vi "ManualAutoScan.vi"(8 "Button-OK":bool, 10 "menu reference":refnum<k9>, 11 "SN Length":string) -> (1 "MainProcess":T1, 3 "Barcode out:":string)   [LabVIEW 2013]
uses:
  Control/SystemProcess.ctl
  Control/Buffer.vi
panel:
  in  "menu reference 2":refnum<k9>
  in  "Button-Cancel":bool
  in  "Barcode(S/N):":string
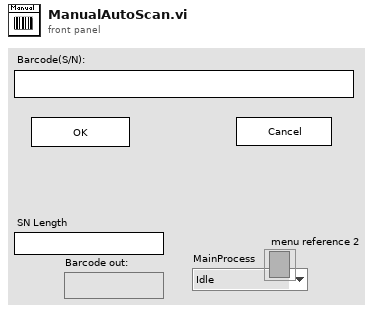
[diagram p1: front panel]
types:
  T1 = typedef "SystemProcess.ctl" = enum16{"Idle", "SystemInit", "SpecialEvent", "Barcode(SN)", "TestInitialize", "Test", "Stop", "SaveTestData", "Exit"}
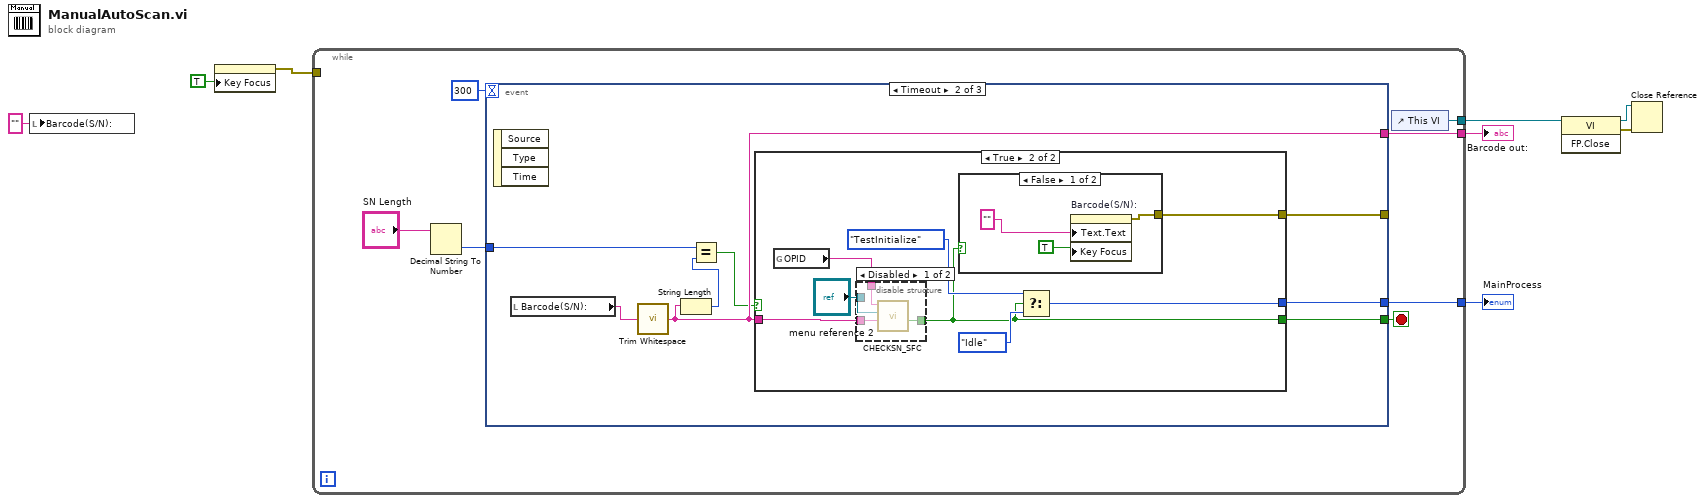
[diagram p0: block diagram]
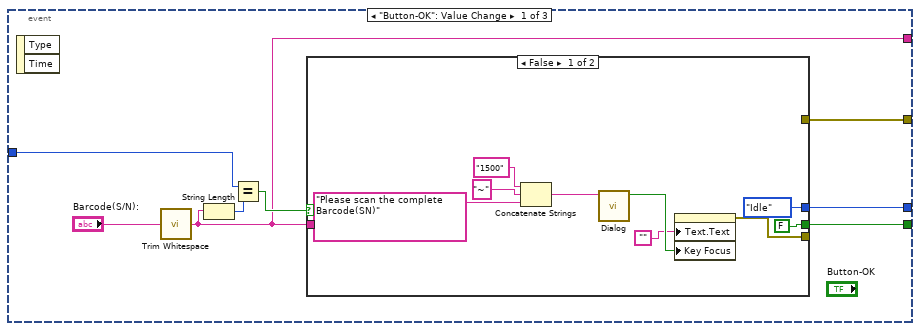
[diagram p2: hidden frame]
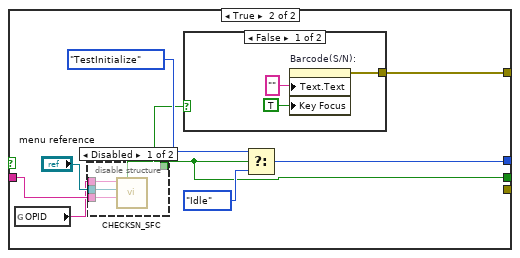
[diagram p3: hidden frame]
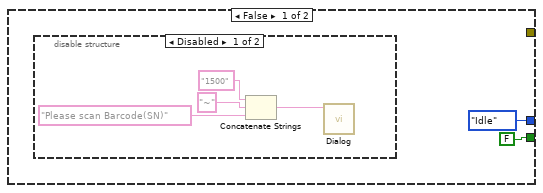
[diagram p6: hidden frame]
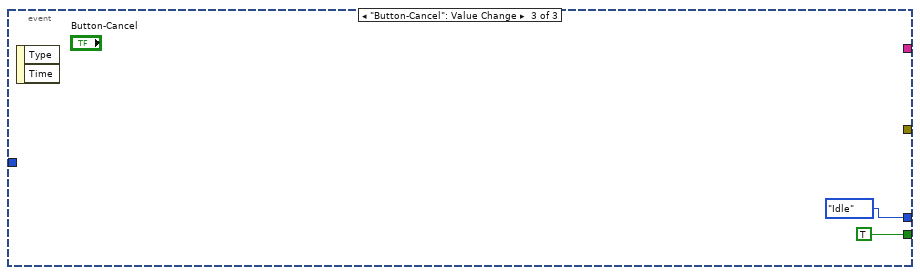
[diagram p10: hidden frame]
diagram:
  n1 = local write "Barcode(S/N):"("" ("Barcode(S/N):")) -> ()
  n2 = property on="Barcode(S/N):" class="Str"("Key Focus"=TRUE) -> (error out=w3:errorcluster)  [unwired: 2 in, 1 out]
  n3 = while {
    tunnel: [w15] -> w5
    tunnel: [w14] -> w4
    tunnel: w3 -> [_]
    tunnel: [w12] -> w2
    stop <- w13 stop-if-true
    n4 = Decimal String To Number(string="SN Length") -> (number=w9:i32)  [unwired: 2 in, 1 out]
    n5 = event shown="[1] Timeout" {
      selector: _ -> [_ _ _]
      dyn-events: _ -> [_ _ _]
      timeout: 300 -> [_ _ _]
      tunnel: [w22 w54 TRUE ("OK in")] -> w13
      tunnel: [w16 w52 _] -> w14
      tunnel: [w23 w55 SystemProcess."Idle" ("MainProcess")] -> w12
      tunnel: [w21 w53 _] -> _
      tunnel: w9 -> [w17 w48 _]
      event "Button-OK": Value Change {
        n6 = event-data() -> ()  [unwired: 1 in, 2 out]
        n7 = call <vilib>:"Trim Whitespace.vi"("string"="Barcode(S/N):") -> ("trimmed string"=w16:string)  [unwired: 1 in]
        n8 = String Length(string=w16) -> (length=w18:i32)
        n9 = Equal?(x=w17, y=w18) -> (x = y?=w19:bool)
        n10 = case shown="False" w19 {
          tunnel: [SystemProcess."Idle" ("MainProcess") w39] -> w23
          tunnel: [FALSE ("OK in") w34] -> w22
          tunnel: [w30 _] -> _
          tunnel: w16 -> [_ w35]
          tunnel: [_ w37] -> w21
          frame False {
            n11 = Concatenate Strings("1500" ("string"), "~" ("string"), "Please scan the complete Barcode(SN)" ("message")) -> (w26:string)
            n12 = call "Dialog.vi"("Limit"=w26) -> ("true"=w25:bool)  [unwired: 9 in, 1 out]
            n13 = property on="Barcode(S/N):" class="Str"("Text.Text"="", "Key Focus"=w25) -> (error out=w30:errorcluster)  [unwired: 2 in, 1 out]
          }
          frame True {
            n14 = global read "Buffer.vi" "OPID"() -> (w33:string)
            n15 = disable-structure shown="Disabled" {
              disable-tunnel: "menu reference" -> [w44 _]
              disable-tunnel: w35 -> [w43 _]
              disable-tunnel: [w42 _] -> w34
              disable-tunnel: w33 -> [w41 _]
              frame Disabled {
                n16 = call "CHECKSN_SFC.vi"("SN"=w43, "menu reference"=w44, "OPID"=w41) -> ("SNCheck"=w42:bool)  [unwired: 7 in, 1 out]
              }
              frame Enabled {
              }
            }
            n17 = case shown="False" w34 {
              tunnel: [w45 _] -> w37
              frame False {
                n18 = property on="Barcode(S/N):" class="Str"("Text.Text"="", "Key Focus"=TRUE) -> (error out=w45:errorcluster)  [unwired: 2 in, 1 out]
              }
              frame True {
              }
            }
            n19 = Select(t=SystemProcess."TestInitialize" ("MainProcess"), s=w34, f=SystemProcess."Idle") -> (s? t:f=w39:T1)
          }
        }
      }
      event Timeout {
        n20 = event-data() -> ()  [unwired: 1 in, 3 out]
        n21 = local read "Barcode(S/N):"() -> (w51:string)
        n22 = call <vilib>:"Trim Whitespace.vi"("string"=w51) -> ("trimmed string"=w52:string)  [unwired: 1 in]
        n23 = String Length(string=w52) -> (length=w50:i32)
        n24 = Equal?(x=w48, y=w50) -> (x = y?=w49:bool)
        n25 = case shown="True" w49 {
          tunnel: [SystemProcess."Idle" ("MainProcess") w67] -> w55
          tunnel: [FALSE ("OK in") w65] -> w54
          tunnel: w52 -> [_ w69]
          tunnel: [_ w64] -> w53
          frame False {
            n26 = disable-structure shown="Disabled" {
              frame Disabled {
                n27 = Concatenate Strings("1500" ("string"), "~" ("string"), "Please scan Barcode(SN)" ("message")) -> (w58:string)
                n28 = call "Dialog.vi"("Limit"=w58) -> ()  [unwired: 9 in, 2 out]
              }
              frame Enabled {
              }
            }
          }
          frame True {
            n29 = global read "Buffer.vi" "OPID"() -> (w62:string)
            n30 = disable-structure shown="Disabled" {
              disable-tunnel: w69 -> [w73 _]
              disable-tunnel: [w72 _] -> w65
              disable-tunnel: "menu reference 2" -> [w71 _]
              disable-tunnel: w62 -> [w70 _]
              frame Disabled {
                n31 = call "CHECKSN_SFC.vi"("SN"=w73, "menu reference"=w71, "OPID"=w70) -> ("SNCheck"=w72:bool)  [unwired: 7 in, 1 out]
              }
              frame Enabled {
              }
            }
            n32 = case shown="False" w65 {
              tunnel: [w76 _] -> w64
              frame False {
                n33 = property on="Barcode(S/N):" class="Str"("Text.Text"="", "Key Focus"=TRUE) -> (error out=w76:errorcluster)  [unwired: 2 in, 1 out]
              }
              frame True {
              }
            }
            n34 = Select(t=SystemProcess."TestInitialize" ("MainProcess"), s=w65, f=SystemProcess."Idle") -> (s? t:f=w67:T1)
          }
        }
      }
      event "Button-Cancel": Value Change {
        n35 = event-data() -> ()  [unwired: 1 in, 2 out]
      }
    }
    n36 = control-ref of="This VI"() -> (w15:refnum<vi>)
  }
  "Barcode out:" <- w4
  "MainProcess" <- w2
  n37 = invoke class="VI" method="FP.Close"(reference=w5) -> (reference out=w7:refnum<vi>, error out=w6:errorcluster)  [unwired: 2 in, 1 out]
  n38 = Close Reference(reference=w7, error in (no error)=w6) -> ()  [unwired: 1 out]
